vi "SLB - Board Power.vi"(0 "GEA2 Reference In":refnum<k24>, 7 "Action":enum16{"Power ON", "Power OFF"}(ring), 11 "Error In":errorcluster) -> (4 "GEA2 Reference Out":refnum<k24>, 6 "Pass/Fail?":bool, 8 "Report Text":string, 15 "Error Out":errorcluster)   [LabVIEW 2016]
doc: "Use this VI to lock or unlock the lid."
uses:
  Q:/Common/DLLs/GEA3/GeaCommunication.dll
  Common/DLLs/GEA3/GeaCommunication.dll
  Common/LabVIEW GEA2 Toolkit/LabVIEW_GEA2_Toolkit.lvlibp/type defs/Source_Destination.ctl
  Common/LabVIEW GEA2 Toolkit/LabVIEW_GEA2_Toolkit.lvlibp/type defs/ERD Read Data In.ctl
  Common/LabVIEW GEA2 Toolkit/LabVIEW_GEA2_Toolkit.lvlibp/type defs/Data Type.ctl
  Common/LabVIEW GEA2 Toolkit/LabVIEW_GEA2_Toolkit.lvlibp
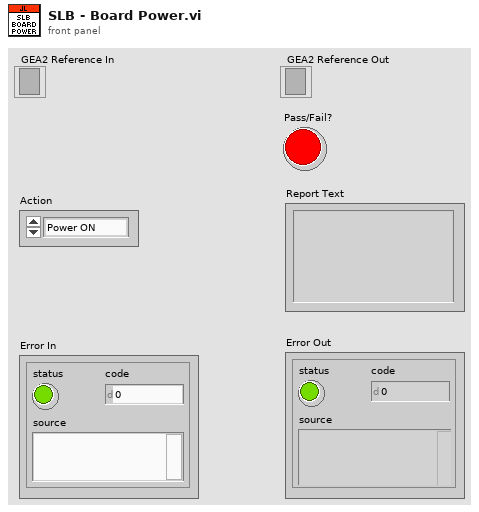
[diagram p1: front panel]
types:
  T1 = typedef "LabVIEW_GEA2_Toolkit.lvlibp/Source_Destination.ctl" = cluster{"Source":u8, "Destination":u8}
  T2 = typedef "LabVIEW_GEA2_Toolkit.lvlibp/ERD Read Data In.ctl" = cluster{"ERD Number":u16, "Data Type":T3}
  T3 = typedef "LabVIEW_GEA2_Toolkit.lvlibp/Data Type.ctl" = enum16{"string", "boolean", "uint8_t", "uint16_t", "uint32_t", "uint64_t", "int8_t", "int16_t", "int32_t", "int64_t"}
  T4 = typedef "LabVIEW_GEA2_Toolkit.lvlibp/ERD Read Data Out.ctl" = cluster{"ERD Number":u16, "Data":string}
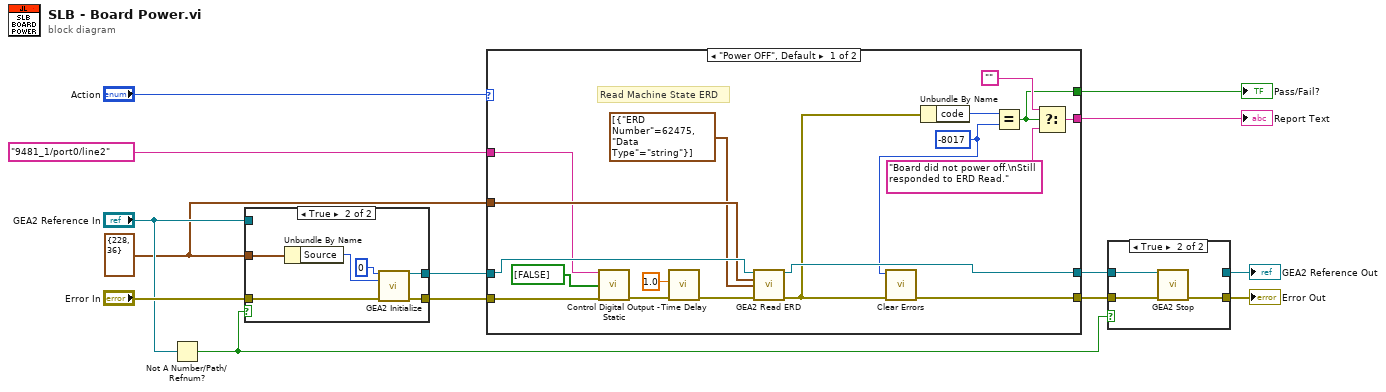
[diagram p0: block diagram]
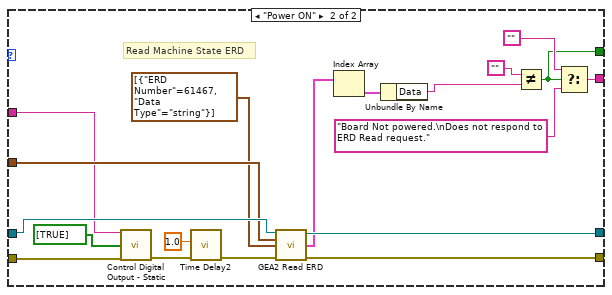
[diagram p2: hidden frame]
diagram:
  w2 = T1 {"Source"=228, "Destination"=36} ("GEA Inputs")
  n1 = Not A Number/Path/Refnum?(number/path/refnum="GEA2 Reference In") -> (NaN/Path/Refnum?=w11:bool)
  n2 = case shown="True" w11 {
    tunnel: "Error In" -> [w15 w22]
    tunnel: [w15 w21] -> w9
    tunnel: "GEA2 Reference In" -> [w16 _]
    tunnel: [w16 w20] -> w7
    tunnel: w2 -> [_ w18]
    frame False {
    }
    frame True {
      n3 = Unbundle By Name(w18) -> ("Source"=w19:u8)
      n4 = call "GEA2 Initialize.vi"("Board Index"=0, "Source Address"=w19, "error in"=w22) -> ("GEA2 Reference Out"=w20:refnum<k24>, "error out"=w21:errorcluster)  [unwired: 10 in, 1 out]
    }
  }
  n5 = case shown="\"Power OFF\", Default" "Action" {
    tunnel: w9 -> [w39 w58]
    tunnel: [w24 w45] -> w8
    tunnel: w7 -> [w38 w57]
    tunnel: [w35 w54] -> w6
    tunnel: [w26 w46] -> w4
    tunnel: [w27 w47] -> w3
    tunnel: w2 -> [w37 w56]
    tunnel: tag "9481_1/port0/line2" ("Line(s)") -> [w34 w53]
    frame "Power OFF", Default {
      w23 = -8017 ("y")
      # "Read Machine State ERD"
      n6 = call "Control Digital Output - Static.vi"("Line(s)"=w34, "Output Array"=bool[] [FALSE], "Error In"=w39) -> ("Error Out"=w32:errorcluster)  [unwired: 12 in]
      n7 = call "Time Delay"("error in (no error)"=w32, "Delay Time (s)"=1.0) -> ("error out"=w31:errorcluster)  [unwired: 9 in]
      n8 = call "GEA2 Read ERD.vi"("GEA2 Reference In"=w38, "GEA Inputs"=w37, "Read ERD List"=T2[] [{"ERD Number"=62475, "Data Type"=enum."string"}], "Error In"=w31) -> ("GEA2 Reference Out"=w35:refnum<k24>, "Error Out"=w25:errorcluster)  [unwired: 8 in, 2 out]
      n9 = call <vilib>:"Clear Errors.vi"("error in (no error)"=w25, "specific error code to clear (0: all)"=w23) -> ("error out"=w24:errorcluster)  [unwired: 4 in, 1 out]
      n10 = Unbundle By Name(w25) -> ("code"=w30:i32)
      n11 = Equal?(x=w30, y=w23) -> (x = y?=w26:bool)
      n12 = Select(t="", s=w26, f="Board did not power off.\nStill responded to ERD Read.") -> (s? t:f=w27:string)
    }
    frame "Power ON" {
      # "Read Machine State ERD"
      n13 = call "Control Digital Output - Static.vi"("Line(s)"=w53, "Output Array"=bool[] [TRUE], "Error In"=w58) -> ("Error Out"=w51:errorcluster)  [unwired: 12 in]
      n14 = call "Time Delay2"("error in (no error)"=w51, "Delay Time (s)"=1.0) -> ("error out"=w50:errorcluster)  [unwired: 9 in]
      n15 = call "GEA2 Read ERD.vi"("GEA2 Reference In"=w57, "GEA Inputs"=w56, "Read ERD List"=T2[] [{"ERD Number"=61467, "Data Type"=enum."string"}], "Error In"=w50) -> ("GEA2 Reference Out"=w54:refnum<k24>, "ERD Data Out"=w44:T4[], "Error Out"=w45:errorcluster)  [unwired: 8 in, 1 out]
      n16 = Index Array(array=w44) -> (element=w43:T4)  [unwired: 1 in]
      n17 = Unbundle By Name(w43) -> ("Data"=w42:string)
      n18 = Not Equal?(x="", y=w42) -> (x != y?=w46:bool)
      n19 = Select(t="", s=w46, f="Board Not powered.\nDoes not respond to ERD Read request.") -> (s? t:f=w47:string)
    }
  }
  "Pass/Fail?" <- w4
  "Report Text" <- w3
  n20 = case shown="True" w11 {
    tunnel: w8 -> [w61 w64]
    tunnel: [w61 w63] -> w14
    tunnel: [w60 _] -> w13
    tunnel: w6 -> [w60 w62]
    frame False {
    }
    frame True {
      n21 = call "GEA2 Stop.vi"("GEA2 Reference In"=w62, "Error In"=w64) -> ("Error Out"=w63:errorcluster)  [unwired: 13 in]
    }
  }
  "Error Out" <- w14
  "GEA2 Reference Out" <- w13
